vi "Clear(SGL).vi"(8 "错误输入":errorcluster) -> (0 "错误输出":errorcluster)   [LabVIEW 2013, in "Tag Data by Variant.lvlib"]
uses:
  Tag Data by Variant.lvlib
  Core/TagVar Data(SGL).vi
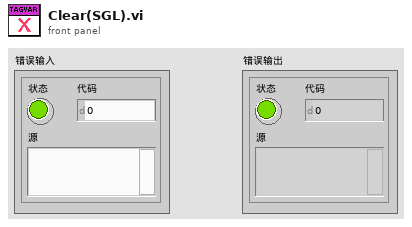
[diagram p1: front panel]
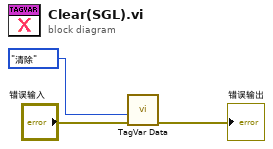
[diagram p0: block diagram]
diagram:
  n1 = call-poly "TagVar Data.vi"("错误输入"="错误输入", "method"=enum16{"初始化", "加入", "删除", "读取", "读取所有", "清除"}."清除") -> ("错误输出"=→"错误输出":errorcluster)  [unwired: 7 in, 2 out]
